vi "Do Not Log Command.vi"(11 "UI Process Command in":refnum<class "Generic UI Process Command.lvclass">) -> (3 "UI Process Command out":refnum<class "Generic UI Process Command.lvclass">)   [LabVIEW 2019, in "User Interface Process.lvlib" / "Generic UI Process Command.lvclass"]
uses:
  Generic UI Process Command.lvclass
  Generic UI Process Command.lvclass/Generic UI Process Command.ctl
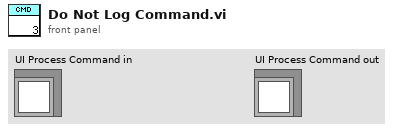
[diagram p1: front panel]
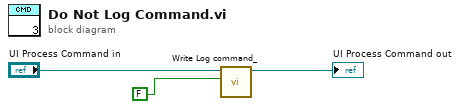
[diagram p0: block diagram]
diagram:
  n1 = call "Write Log command_.vi"("Log command?"=FALSE, "Generic UI Process Command in"="UI Process Command in") -> ("Generic UI Process Command out"=→"UI Process Command out":refnum<class "Generic UI Process Command.lvclass">)  [unwired: 9 in]
